vi "Write.vi"(9 "timeout in ms (-1)":i32, 10 "Element":T1, 11 "Enclave in":refnum<class "Enclave.lvclass">) -> (1 "timed out?":bool, 4 "Closed?":bool)   [LabVIEW 2022 SP3, in "Enclave.lvlib" / "Enclave.lvclass"]
uses:
  Enclave.lvclass
  Element.ctl
  Enclave.lvclass/Enclave.ctl
  Enclave Event.ctl
  Enclave.lvlib
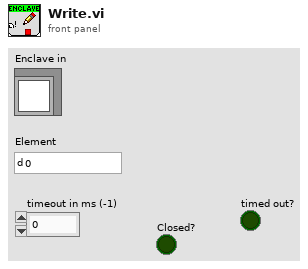
[diagram p1: front panel]
types:
  T1 = typedef "Enclave.lvlib/Element.ctl" = dbl
  T2 = typedef "Enclave.lvlib/Writer Data.ctl" = cluster{"Queues":refnum<queue>[], "Lossy":bool, "Event":bool}
  T3 = typedef "Enclave.lvlib/Tag Data.ctl" = cluster{"Element":T1, "Sequence":u64, "Time Stamp":timestamp}
  T4 = typedef "Enclave.lvlib/Enclave Event.ctl" = cluster{"Element":T1, "Closed":bool}
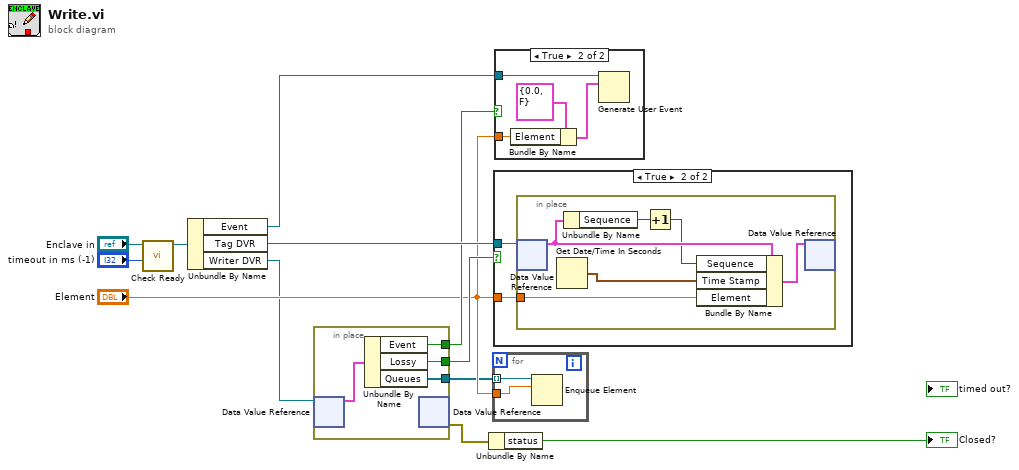
[diagram p0: block diagram]
diagram:
  n1 = call "Check Ready.vi"("Timeout"="timeout in ms (-1)", "Enclave in"="Enclave in") -> ("Enclave out"=w7:refnum<class "Enclave.lvclass">)  [unwired: 7 in, 2 out]
  n2 = Unbundle By Name(w7) -> ("Event"=w4:refnum<user-event>, "Tag DVR"=w11:refnum<data-value>, "Writer DVR"=w5:refnum<data-value>)
  n3 = in-place {
    in-place-border: [w15] -> w3
    in-place-border: [w14] -> w12
    in-place-border: [w13] -> w10
    n4 = in-place-dvr #1(w5) -> (w16:T2)  [unwired: 1 out]
    n5 = Unbundle By Name(w16) -> ("Event"=w13:bool, "Lossy"=w14:bool, "Queues"=w15:refnum<queue>[])
    n6 = in-place-dvr #1() -> (w2:errorcluster)  [unwired: 1 in, 1 out]
  }
  n7 = Unbundle By Name(w2) -> ("status"=→"Closed?":bool)
  n8 = for {
    tunnel: w3 -> [w18] mode=indexing
    tunnel: "Element" -> [w17]
    n9 = Enqueue Element(queue=w18, element=w17) -> ()  [unwired: 2 in, 3 out]
  }
  n10 = case shown="True" w12 {
    tunnel: w11 -> [_ w20]
    tunnel: "Element" -> [_ w19]
    frame False {
    }
    frame True {
      n11 = in-place {
        in-place-border: w19 -> [w24]
        n12 = in-place-dvr #2(w20) -> (w25:T3)  [unwired: 1 out]
        n13 = Get Date/Time In Seconds() -> (seconds since 1Jan1904=w23:timestamp)
        n14 = Unbundle By Name(w25) -> ("Sequence"=w26:u64)
        n15 = Increment(x=w26) -> (x+1=w21:u64)
        n16 = Bundle By Name(cluster=w25, "Sequence"=w21, "Time Stamp"=w23, "Element"=w24) -> (w22:T3)
        n17 = in-place-dvr #2(w22) -> ()  [unwired: 2 out]
      }
    }
  }
  n18 = case shown="True" w10 {
    tunnel: w4 -> [_ w30]
    tunnel: "Element" -> [_ w27]
    frame False {
    }
    frame True {
      n19 = Bundle By Name(cluster=T4 {"Element"=0.0, "Closed"=FALSE} ("event data"), "Element"=w27) -> (w28:T4)
      n20 = Generate User Event(user event=w30, event data cluster=w28) -> ()  [unwired: 2 in, 2 out]
    }
  }
